vi "Motor Multiplexer-Remote.vi"() -> ()   [LabVIEW 2009]
uses:
  <vilib>/NXT/Subs/LVHSConnector.ctl
  <vilib>/NXT/Block Support/NXT_InputPort.ctl
panel:
  in  "Direction":bool
  in  "Power":u8=100 max=100 step=1
  in  "Mode":u8(ring)=1 items=["RUN", "FLT", "BRK"]
  in  "Motor":u8=1 min=1 max=4 step=1
  out "Status":bool caption="Success?"
  in  "Input Port":T1 items=["Port 1", "Port 2", "Port 3", "Port 4"]
  in  "NXT":T2
  out "NXT dup":T2 caption="NXT"
  # "mindsensors.com\nCopyright (c) 2009 by mindsensors.com\nEmail: info (<at>) mindsensors (<dot>) com\n\nThis program is free software. You can redistribute it and/or modify\nit under the terms of the GNU General Public License as published by\nthe Free Software Foundation; version 3 of the License.\nRead the license at: http://www.gnu.org/licenses/gpl.txt"
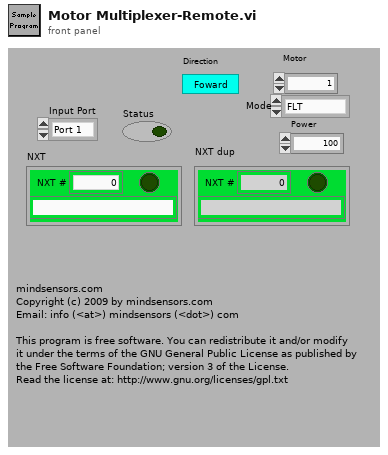
[diagram p1: front panel]
types:
  T1 = typedef "NXT_InputPort.ctl" = u8
  T2 = typedef "LVHSConnector.ctl" = cluster{"error":errorcluster, "address":string, "NXT #":i32, "Show Error":bool}
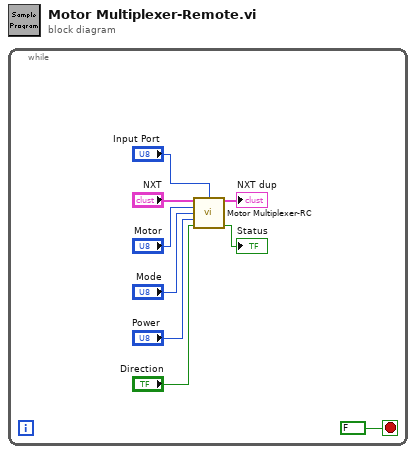
[diagram p0: block diagram]
diagram:
  n1 = while {
    stop <- FALSE stop-if-true
    n2 = call "Motor Multiplexer-RC.vi"("NXT"="NXT", "Input Port"="Input Port", "Motor"="Motor", "Mode"="Mode", "Power"="Power", "Direction"="Direction") -> ("NXT dup"=→"NXT dup":T2, "Status"=→"Status":bool)  [unwired: 8 in]
  }
